vi "Create Filename.vi"(7 "Sensor SN":string, 11 "Logging Configuration":T1) -> (3 "appended path":path)   [LabVIEW 2018, in "Logging.lvlib"]
uses:
  Logging.lvlib
  Logging Configuration.ctl
  <vilib>/addons/database/Connection.llb/Conn ObjectReference.ctl
  <vilib>/addons/database/NI_Database_API.lvlib
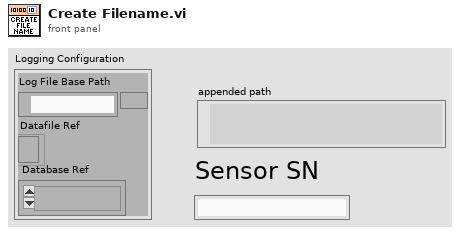
[diagram p1: front panel]
types:
  T1 = typedef "Logging.lvlib/Logging Configuration.ctl" = cluster{"Log File Base Path":path, "Datafile Ref":refnum<file>, "Database Ref":T2}
  T2 = typedef "NI_Database_API.lvlib/Conn ObjectReference.ctl" = refnum<k1>
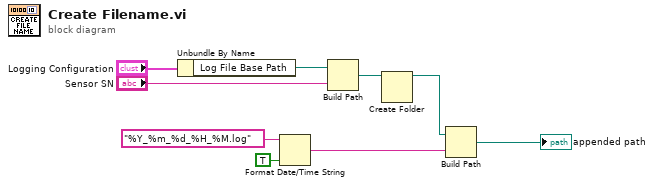
[diagram p0: block diagram]
diagram:
  n1 = Unbundle By Name("Logging Configuration") -> ("Log File Base Path"=w3:path)
  n2 = Format Date/Time String(time format string (%c)="%Y_%m_%d_%H_%M.log", UTC format=TRUE) -> (date/time string=w6:string)  [unwired: 1 in]
  n3 = Build Path(base path=w3, name or relative path="Sensor SN") -> (appended path=w2:path)
  n4 = Create Folder(path (use dialog)=w2) -> (created path=w1:path)  [unwired: 2 in, 2 out]
  n5 = Build Path(base path=w1, name or relative path=w6) -> (appended path=→"appended path":path)
